vi "SetColor.vi"(8 "error in (no error)":errorcluster, 10 "Color":refnum<class "Color.lvclass">, 11 "Point in":refnum<class "PointSpecialized.lvclass">) -> (0 "error out":errorcluster, 3 "Point out":refnum<class "PointSpecialized.lvclass">)   [LabVIEW 2021, in "Picture2D.lvlib" / "PointSpecialized.lvclass"]
uses:
  PointSpecialized.lvclass
  Color/Color.lvclass
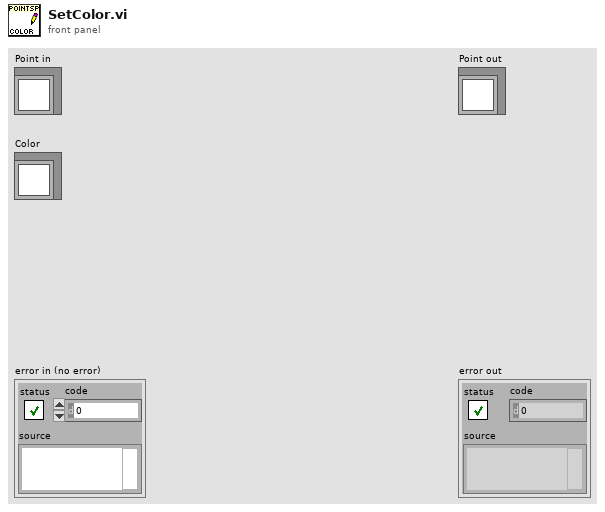
[diagram p1: front panel]
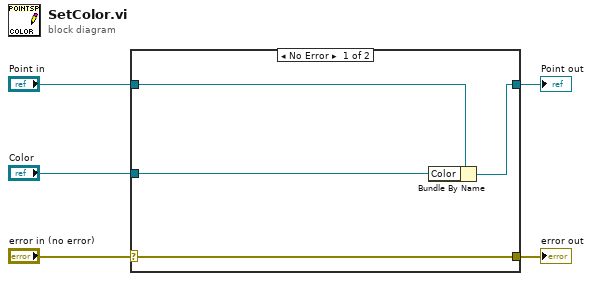
[diagram p0: block diagram]
diagram:
  n1 = case shown="No Error" "error in (no error)" {
    selector: "error in (no error)" -> [w9 w10]
    tunnel: [w9 w10] -> w4
    tunnel: [w7 w11] -> w2
    tunnel: "Point in" -> [w8 w11]
    tunnel: "Color" -> [w6 _]
    frame No Error {
      n2 = Bundle By Name(cluster=w8, "Color"=w6) -> (w7:refnum<class "PointSpecialized.lvclass">)
    }
    frame Error {
    }
  }
  "error out" <- w4
  "Point out" <- w2
